vi "Read NChan NSamp 2D SGL.vi"(8 "error in (no error)":errorcluster, 9 "timeout [s]":dbl=-1.0, 10 "number of samples per channel":i32=1000, 11 "MicroDAQ.lvlib:Analog Input.lvclass":refnum<class "Analog Input.lvclass">) -> (0 "error out":errorcluster, 1 "read samples":i32, 2 "Values":dbl[][](array[numeric]), 3 "MicroDAQ.lvlib:Analog Input.lvclass out":refnum<class "Analog Input.lvclass">)   [LabVIEW 2009, in "MicroDAQ.lvlib" / "Analog Input.lvclass"]
doc: "Reads a buffor of floating-point samples from each channel."
uses:
  <instrlib>/MicroDAQ/Channel/Analog Input/Analog Input.lvclass
  <instrlib>/MicroDAQ/Channel/Analog Input/Analog Input.lvclass/Analog Input.ctl
  <instrlib>/MicroDAQ/Mlink library wraper/mlink.lvlib
  <instrlib>/MicroDAQ/Channel/Channel.lvclass
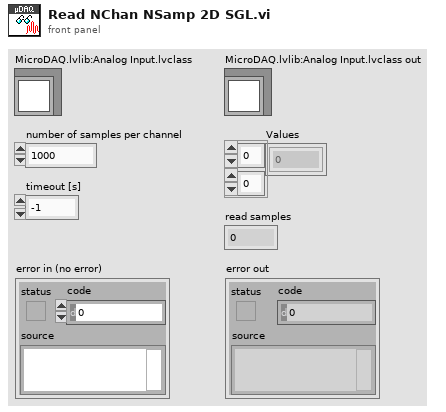
[diagram p1: front panel]
types:
  T1 = typedef "MicroDAQ.lvlib/Analog input Channel enum.ctl" = u16
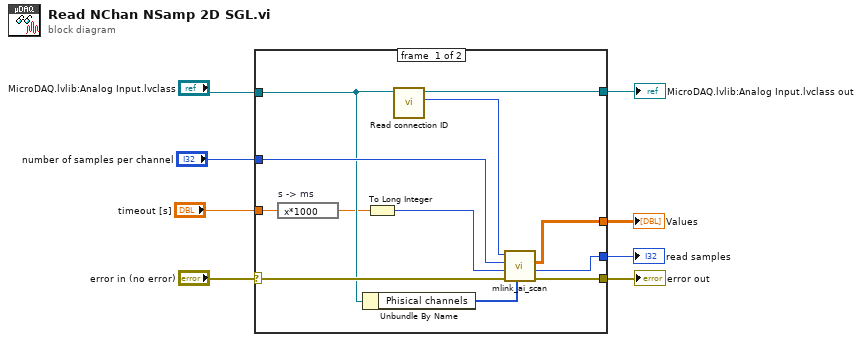
[diagram p0: block diagram]
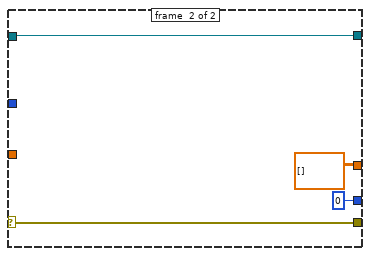
[diagram p2: hidden frame]
diagram:
  n1 = case shown="No Error" "error in (no error)" {
    selector: "error in (no error)" -> [w20 w23]
    tunnel: [w19 w23] -> w7
    tunnel: [w17 w24] -> w6
    tunnel: "number of samples per channel" -> [w16 _]
    tunnel: "MicroDAQ.lvlib:Analog Input.lvclass" -> [w13 w24]
    tunnel: [w14 0 ("read samples")] -> w3
    tunnel: [w12 dbl[][] [] ("Values")] -> w2
    tunnel: "timeout [s]" -> [w11 _]
    frame #0 {
      n2 = expression code="x*1000" "s -> ms"(w11) -> (w10:dbl)
      n3 = Unbundle By Name(w13) -> ("Phisical channels"=w15:T1[])
      n4 = To Long Integer(number=w10) -> (32bit integer=w9:i32)
      n5 = call <instrlib>:"Read connection ID.vi"("Task in"=w13) -> ("connection ID"=w18:i32, "Task out"=w17:refnum<class "Analog Input.lvclass">)  [unwired: 9 in]
      n6 = call <instrlib>:"mlink_ai_scan .vi"("Channels"=w15, "error in (no error)"=w20, "timeout"=w9, "scan count"=w16, "connection ID"=w18) -> ("error out"=w19:errorcluster, "read samples"=w14:i32, "Values"=w12:dbl[][])  [unwired: 3 in, 1 out]
    }
    frame #1 {
    }
  }
  "error out" <- w7
  "MicroDAQ.lvlib:Analog Input.lvclass out" <- w6
  "read samples" <- w3
  "Values" <- w2
